vi "parse_parameters.vi"(3 "error in":errorcluster) -> (0 "error out":errorcluster, 1 "Time control parameters":T1 {"Measurment time interval" format="%.2e"}, 2 "Temp control parameters":T2 {"End Temp" format="%.2f"; "Temp Step" format="%.2f"; "Start Temp" format="%.2f"})   [LabVIEW 2016]
doc: "Opens a file from the path input and reads a text header then build temp control and time control parameters.\n\nMuhannad Alghamdi\nAssignment 4\nCSUSB Physics 350"
uses:
  typedefs/temp_control_params.ctl
  typedefs/time_control_params.ctl
panel:
  out "Path":path
  out "Auto launch data viewer at end":bool
  # "Muhannad Alghamdi\nCSUSB Physics 350"
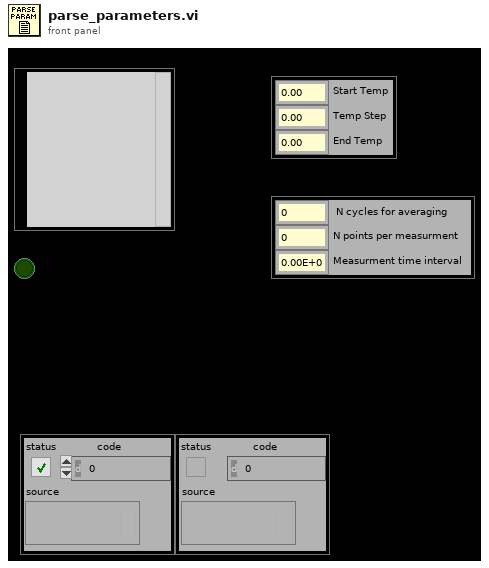
[diagram p1: front panel]
types:
  T1 = typedef "time_control_params.ctl" = cluster{"N cycles for averaging":i32, "N points per measurment":i32, "Measurment time interval":dbl}
  T2 = typedef "temp_control_params.ctl" = cluster{"Start Temp":dbl, "Temp Step":dbl, "End Temp":dbl}
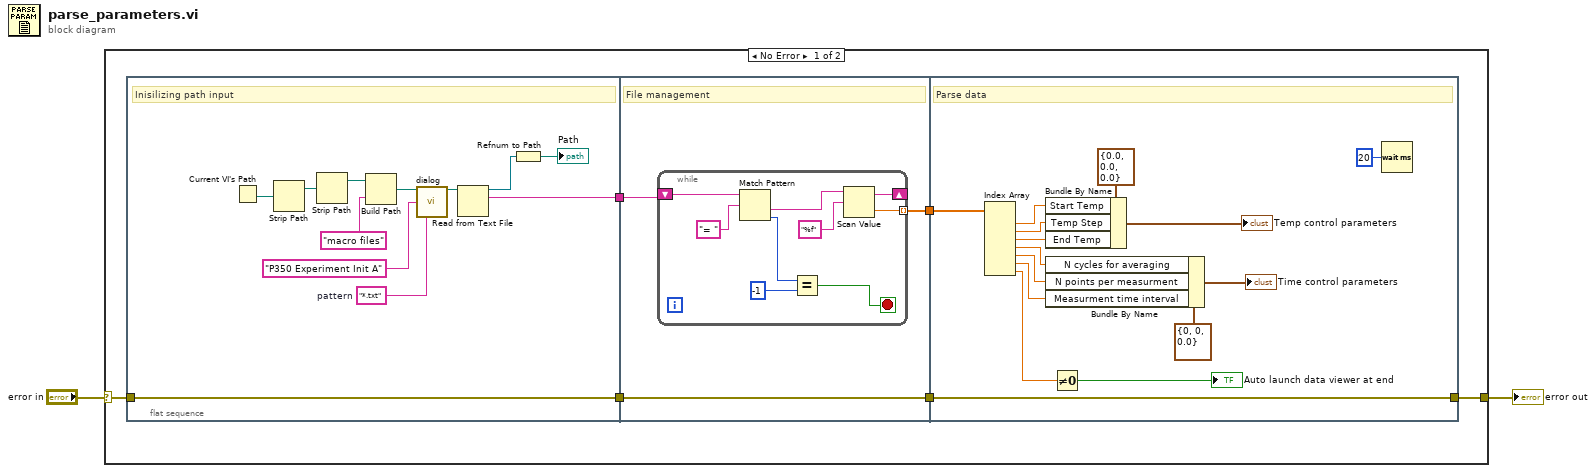
[diagram p0: block diagram]
diagram:
  n1 = case shown="No Error" "error in" {
    selector: "error in" -> [w6 w48]
    tunnel: [w3 w48] -> w1
    frame No Error {
      n2 = flat-sequence {
        tunnel: [w12] -> w8
        tunnel: w6 -> [w9]
        tunnel: [w9] -> w4
        tunnel: [w23] -> w7
        tunnel: w8 -> [w22]
        tunnel: [w21] -> w5
        tunnel: w4 -> [w21]
        tunnel: w7 -> [w47]
        tunnel: [w33] -> w3
        tunnel: w5 -> [w33]
        frame #0 {
          w19 = "*.txt"  # pattern
          # "Inisilizing path input"
          n3 = Current VI's Path() -> (path=w13:path)
          n4 = Strip Path(path=w13) -> (stripped path=w10:path)  [unwired: 1 out]
          n5 = Strip Path(path=w10) -> (stripped path=w11:path)  [unwired: 1 out]
          n6 = Build Path(base path=w11, name or relative path="macro files") -> (appended path=w17:path)
          n7 = call "dialog.vi"("start path"=w17, "default name"="P350 Experiment Init A" ("prompt"), "pattern (all files)"=w19) -> ("selected path"=w18:path)  [unwired: 9 in, 3 out]
          n8 = Read from Text File(file (use dialog)=w18) -> (refnum out=w15:refnum<file>, text=w12:string)  [unwired: 3 in, 2 out]
          n9 = Refnum to Path(1:w15) -> (0:→"Path":path)
        }
        frame #1 {
          # "File management"
          n10 = while {
            shift-right: [w28] -> _
            shift-left: w22 -> [w29]
            tunnel: [w27] -> w23 mode=indexing
            stop <- w24 stop-if-true
            n11 = Match Pattern(string=w29, regular expression="= ") -> (after substring=w31:string, offset past match=w25:i32)  [unwired: 1 in, 2 out]
            n12 = Equal?(x=w25, y=-1) -> (x = y?=w24:bool)
            n13 = Scan Value(string=w31, format string="%f") -> (output string=w28:string, value=w27:dbl)  [unwired: 1 in]
          }
        }
        frame #2 {
          # "Parse data"
          n14 = Index Array(array=w47) -> (element #1=w37:dbl, element #2=w39:dbl, element #3=w42:dbl, element #4=w43:dbl, element #5=w44:dbl, element #6=w45:dbl, element #7=w46:dbl)  [unwired: 7 in]
          n15 = Bundle By Name(cluster=T2 {"Start Temp"=0.0, "Temp Step"=0.0, "End Temp"=0.0} ("temp control parameters"), "Start Temp"=w37, "Temp Step"=w39, "End Temp"=w42) -> (→"Temp control parameters":T2)
          n16 = Bundle By Name(cluster=T1 {"N cycles for averaging"=0, "N points per measurment"=0, "Measurment time interval"=0.0} ("time control parameters"), "N cycles for averaging"=w43, "N points per measurment"=w44, "Measurment time interval"=w45) -> (→"Time control parameters":T1)
          n17 = Not Equal To 0?(x=w46) -> (x != 0?=→"Auto launch data viewer at end":bool)
          n18 = Wait (ms)(milliseconds to wait=u32 20) -> ()  [unwired: 1 out]
        }
      }
    }
    frame Error {
    }
  }
  "error out" <- w1
